vi "Get Unique Directory.vi"(8 "Error In":errorcluster, 10 "Root Folder Name":string="BeagleBone Black", 11 "Parent Directory":path) -> (0 "Error Out":errorcluster, 3 "Target Directory":path)   [LabVIEW 2014, in "LMH-LINX.lvlib"]
uses:
  LMH-LINX.lvlib
  <vilib>/regexp/Match Regular Expression.xnode
  <vilib>/MakerHub/Toolbox/LMH-Toolbox.lvlib
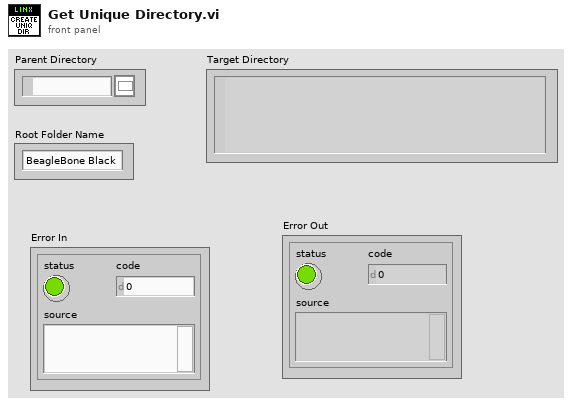
[diagram p1: front panel]
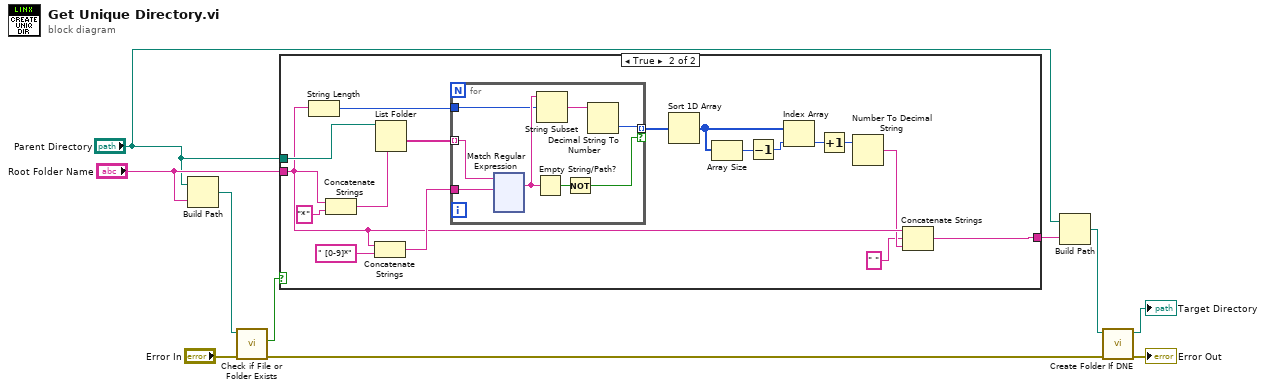
[diagram p0: block diagram]
diagram:
  n1 = Build Path(base path="Parent Directory", name or relative path="Root Folder Name") -> (appended path=w10:path)
  n2 = call <vilib>:"Check if File or Folder Exists.vi"("error in (no error)"="Error In", "path"=w10) -> ("error out"=w3:errorcluster, "file or folder exists?"=w8:bool)  [unwired: 7 in, 1 out]
  n3 = case shown="True" w8 {
    tunnel: [w11 w19] -> w6
    tunnel: "Parent Directory" -> [_ w18]
    tunnel: "Root Folder Name" -> [w11 w16]
    frame False {
    }
    frame True {
      n4 = String Length(string=w16) -> (length=w22:i32)
      n5 = Concatenate Strings(w16, "*" ("string")) -> (w25:string)
      n6 = Concatenate Strings(w16, " [0-9]*" ("string")) -> (w23:string)
      n7 = List Folder(path=w18, pattern=w25) -> (folder names=w21:string[])  [unwired: 1 in, 4 out]
      n8 = for {
        tunnel: w21 -> [w36] mode=indexing
        tunnel: w23 -> [w35]
        tunnel: [w29] -> w20 mode=indexing if=w31
        tunnel: w22 -> [w32]
        n9 = xnode "Match Regular Expression"("input string"=w36, "regular expression"=w35) -> ("whole match"=w33:string)  [unwired: 4 in, 4 out]
        n10 = Empty String/Path?(string/path=w33) -> (empty?=w34:bool)
        n11 = String Subset(string=w33, offset (0)=w32) -> (substring=w30:string)  [unwired: 1 in]
        n12 = Not(x=w34) -> (.not. x?=w31:bool)
        n13 = Decimal String To Number(string=w30) -> (number=w29:i32)  [unwired: 2 in, 1 out]
      }
      n14 = Sort 1D Array(array=w20) -> (sorted array=w13:i32[])
      n15 = Array Size(array=w13) -> (size(s)=w27:i32)
      n16 = Decrement(x=w27) -> (x-1=w26:i32)
      n17 = Index Array(array=w13, index=w26) -> (element=w12:i32)
      n18 = Increment(x=w12) -> (x+1=w17:i32)
      n19 = Number To Decimal String(number=w17) -> (decimal integer string=w15:string)  [unwired: 1 in]
      n20 = Concatenate Strings(w16, " " ("string"), w15) -> (w19:string)
    }
  }
  n21 = Build Path(base path="Parent Directory", name or relative path=w6) -> (appended path=w5:path)
  n22 = call <vilib>:"Create Folder If DNE.vi"("Error In"=w3, "Folder Path"=w5) -> ("Error Out"=→"Error Out":errorcluster, "Dup Path"=→"Target Directory":path)  [unwired: 8 in]
